vi "worksheet filter list.vi"(8 "error in (no error)":errorcluster, 9 "list":u32, 10 "col":u16, 11 "worksheet":u32) -> (0 "error out":errorcluster, 3 "function return":u32(ring))   [LabVIEW 2015, in "xlsxwriter.lvlib"]
doc: "lxw_error worksheet_filter_list(lxw_worksheet worksheet, lxw_col_t col, unsigned long list);"
uses:
  xlsxwriter.lvlib
  xlsxwriter.dll
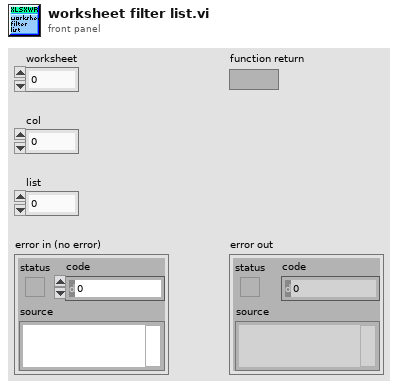
[diagram p1: front panel]
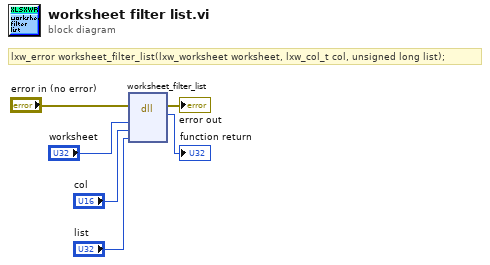
[diagram p0: block diagram]
diagram:
  # "lxw_error worksheet_filter_list(lxw_worksheet worksheet, lxw_col_t col, unsigned long list);"
  n1 = dll-call lib="C:/Users/WDAGUtilityAccount/Desktop/lv_vis_added_cell/xlsxwriter.*" fn="worksheet_filter_list"(error in="error in (no error)", "worksheet"="worksheet", "col"="col", "list"="list") -> (error out=→"error out":errorcluster, →"function return":u32)  [unwired: 5 in, 1 out]
